vi "Psychophysics.vi"() -> ()   [LabVIEW 2017]
panel:
  in  "stop":bool
  out "Generates Random Y":dbl
  out "Generates Random X":dbl
  out "XY Graph":cluster{dbl[], dbl[]}[](graph)
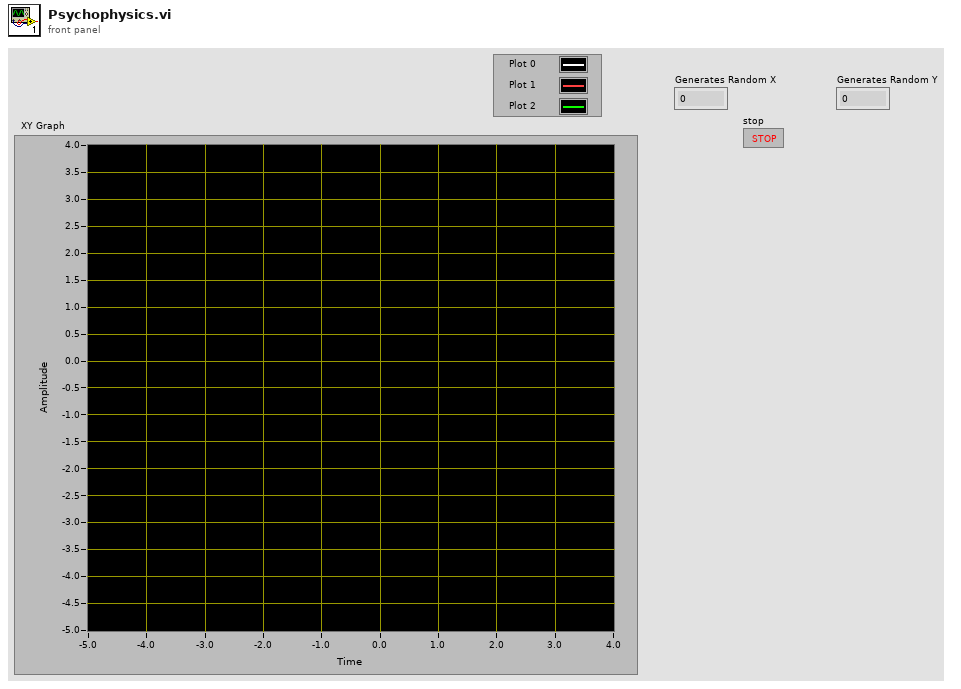
[diagram p1: front panel]
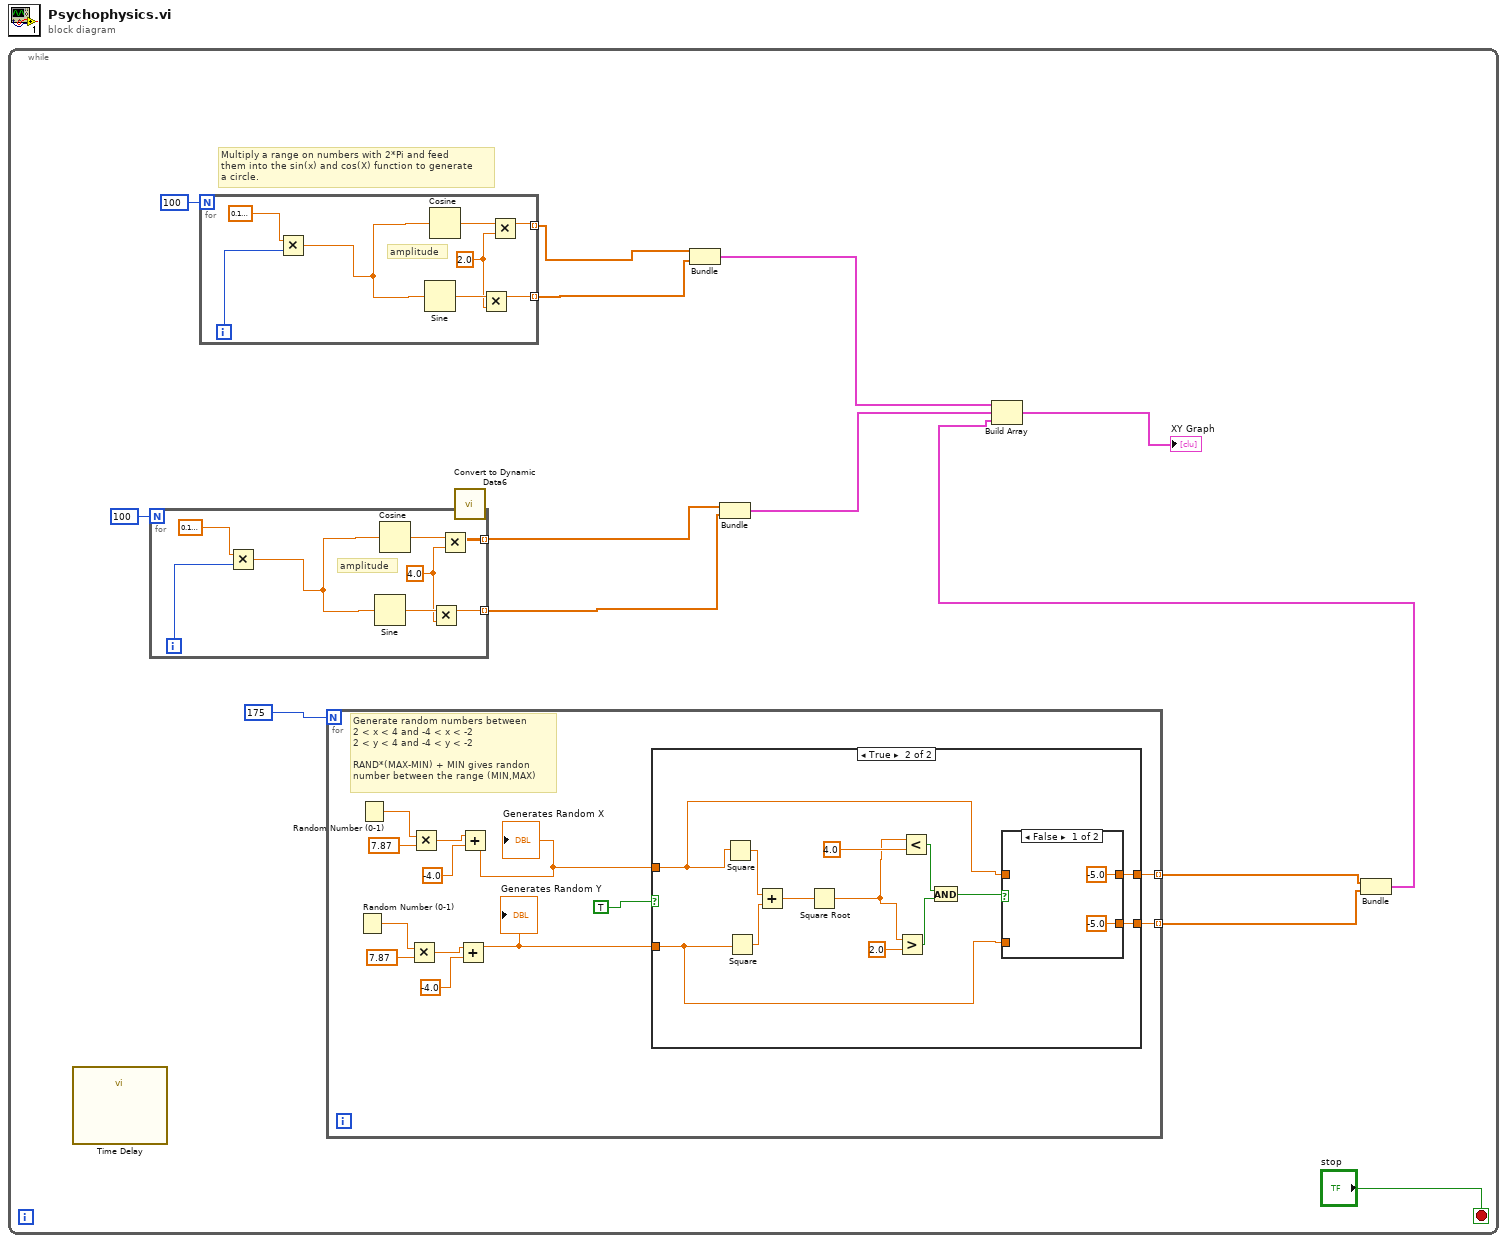
[diagram p0: block diagram]
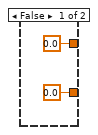
[diagram p2: hidden frame]
diagram:
  n1 = while {
    stop <- "stop" stop-if-true
    # "Multiply a range on numbers with 2*Pi and feed\nthem into the sin(x) and cos(X) function to generate\na circle."
    n2 = call "Time Delay"() -> ()  [unwired: 11 in, 1 out]
    n3 = for {
      N: 100 -> [_]
      tunnel: [w49] -> w7 mode=indexing
      tunnel: [w48] -> w6 mode=indexing
      i -> [w52]
      w47 = sgl 4.0 ("y")
      # "amplitude"
      n4 = Multiply(x=sgl 0.1, y=w52) -> (x*y=w51:sgl)
      n5 = Sine(x=w51) -> (sin(x)=w53:sgl)
      n6 = Cosine(x=w51) -> (cos(x)=w54:sgl)
      n7 = Multiply(x=w53, y=w47) -> (x*y=w48:sgl)
      n8 = Multiply(x=w54, y=w47) -> (x*y=w49:sgl)
    }
    n9 = for {
      N: 100 -> [_]
      tunnel: [w57] -> w9 mode=indexing
      tunnel: [w56] -> w8 mode=indexing
      i -> [w60]
      w55 = sgl 2.0 ("y")
      # "amplitude"
      n10 = Multiply(x=sgl 0.1, y=w60) -> (x*y=w59:sgl)
      n11 = Sine(x=w59) -> (sin(x)=w61:sgl)
      n12 = Cosine(x=w59) -> (cos(x)=w62:sgl)
      n13 = Multiply(x=w61, y=w55) -> (x*y=w56:sgl)
      n14 = Multiply(x=w62, y=w55) -> (x*y=w57:sgl)
    }
    n15 = for {
      N: 175 -> [_]
      tunnel: [w16] -> w10 mode=indexing
      tunnel: [w15] -> w11 mode=indexing
      # "Generate random numbers between \n2 < x < 4 and -4 < x < -2\n2 < y < 4 and -4 < y < -2\n\nRAND*(MAX-MIN) + MIN gives randon\nnumber between the range (MIN,MAX)"
      n16 = Random Number (0-1)() -> (number: 0 to 1=w23:dbl)
      n17 = Random Number (0-1)() -> (number: 0 to 1=w27:dbl)
      n18 = Multiply(x=w23, y=7.87) -> (x*y=w21:dbl)
      n19 = Multiply(x=w27, y=7.87) -> (x*y=w25:dbl)
      n20 = Add(x=w21, y=-4.0) -> (x+y=w18:dbl)
      "Generates Random Y" <- w18
      n21 = Add(x=w25, y=-4.0) -> (x+y=w19:dbl)
      "Generates Random X" <- w19
      n22 = case shown="True" TRUE {
        tunnel: w19 -> [_ w30]
        tunnel: w18 -> [_ w31]
        tunnel: [0.0 w33] -> w16
        tunnel: [0.0 w32] -> w15
        frame False {
        }
        frame True {
          n23 = Square(x=w30) -> (x^2=w42:dbl)
          n24 = Square(x=w31) -> (x^2=w41:dbl)
          n25 = Add(x=w42, y=w41) -> (x+y=w40:dbl)
          n26 = Square Root(x=w40) -> (sqrt(x)=w34:dbl)
          n27 = Greater?(x=w34, y=2.0) -> (0:w36:bool)
          n28 = Less?(x=w34, y=4.0) -> (x < y?=w37:bool)
          n29 = And(x=w37, y=w36) -> (x .and. y?=w35:bool)
          n30 = case shown="False" w35 {
            tunnel: w31 -> [_ w46]
            tunnel: w30 -> [_ w45]
            tunnel: [-5.0 w46] -> w33
            tunnel: [-5.0 w45] -> w32
            frame False {
            }
            frame True {
            }
          }
        }
      }
    }
    n31 = call "Convert to Dynamic Data6"() -> ()  [unwired: 4 in, 1 out]
    n32 = Bundle(w9, w8) -> (w4:cluster{sgl[], sgl[]})  [unwired: 1 in]
    n33 = Bundle(w7, w6) -> (w5:cluster{sgl[], sgl[]})  [unwired: 1 in]
    n34 = Bundle(w11, w10) -> (w2:cluster{dbl[], dbl[]})  [unwired: 1 in]
    n35 = Build Array(w4, w5, w2) -> (→"XY Graph":cluster{dbl[], dbl[]}[])
  }
